vi "实验数据至图表转换.vi"() -> ()   [LabVIEW 2019]
uses:
  <vilib>/Utility/miscctls.llb/LVDateTimeRec.ctl
  <vilib>/Utility/file.llb/Read Delimited Spreadsheet (string).vi
  <vilib>/Utility/NIReport.llb/NI_report.lvclass
  <vilib>/addons/_office/NI_ReportGenerationToolkit.lvlib
  <vilib>/addons/_office/excel.llb/Excel Get Data ([str]).vi
  <vilib>/Utility/NIReport.llb/Excel/NI_Excel.lvclass
panel:
  out "时间标识":timestamp
  in  "template (empty)":path caption="模板（空）"
  out "输入+ 2":cluster{"X":dbl[], "Y":dbl[]}[](graph)
  out "电池+铜排":cluster{"X":dbl[], "Y":dbl[]}[](graph)
  in  "file path (dialog if empty)":path=path "f:/Users/black/Desktop/新建文本文档.txt"
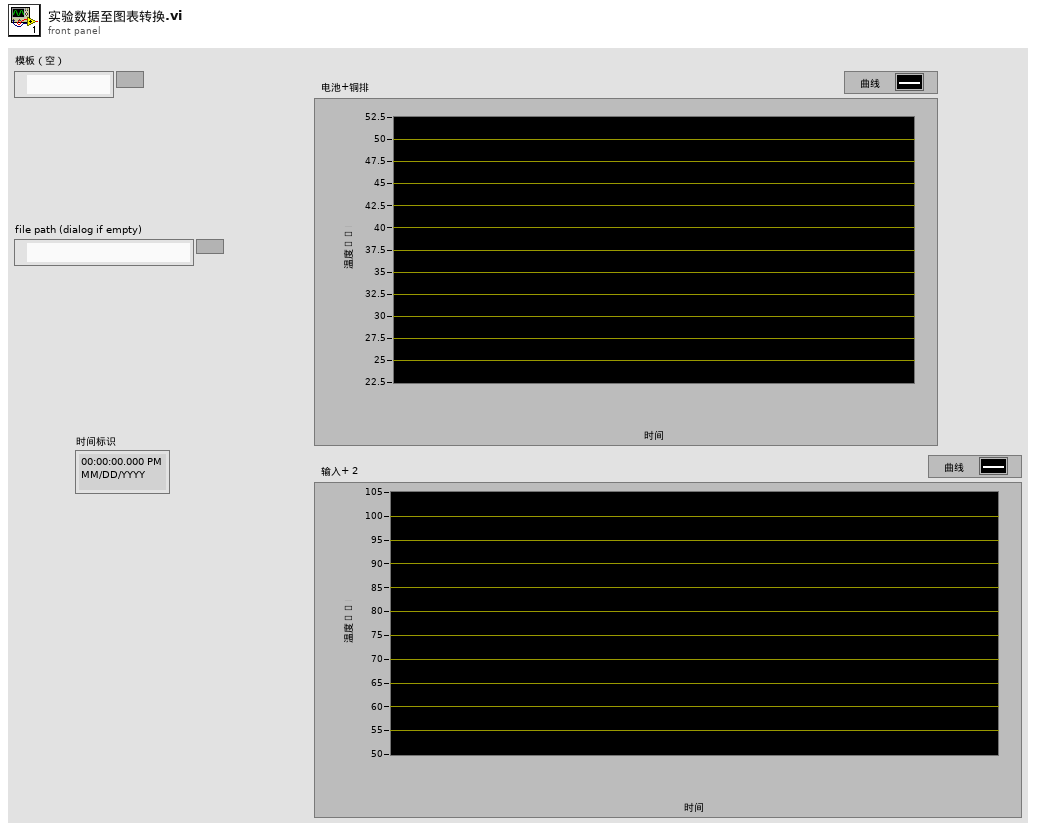
[diagram p1: front panel]
types:
  T1 = typedef "LVDateTimeRec.ctl" = cluster{"fractional second":dbl, "second":i32, "minute":i32, "hour":i32, "day of month":i32, "month":i32, "year":i32, "day of week":i32, "day of year":i32, "DST":i32}
  T2 = enum16{"Standard Report", "HTML", "Word", "Excel"}
  T3 = enum16{"maximized", "minimized", "normal", "no change"}
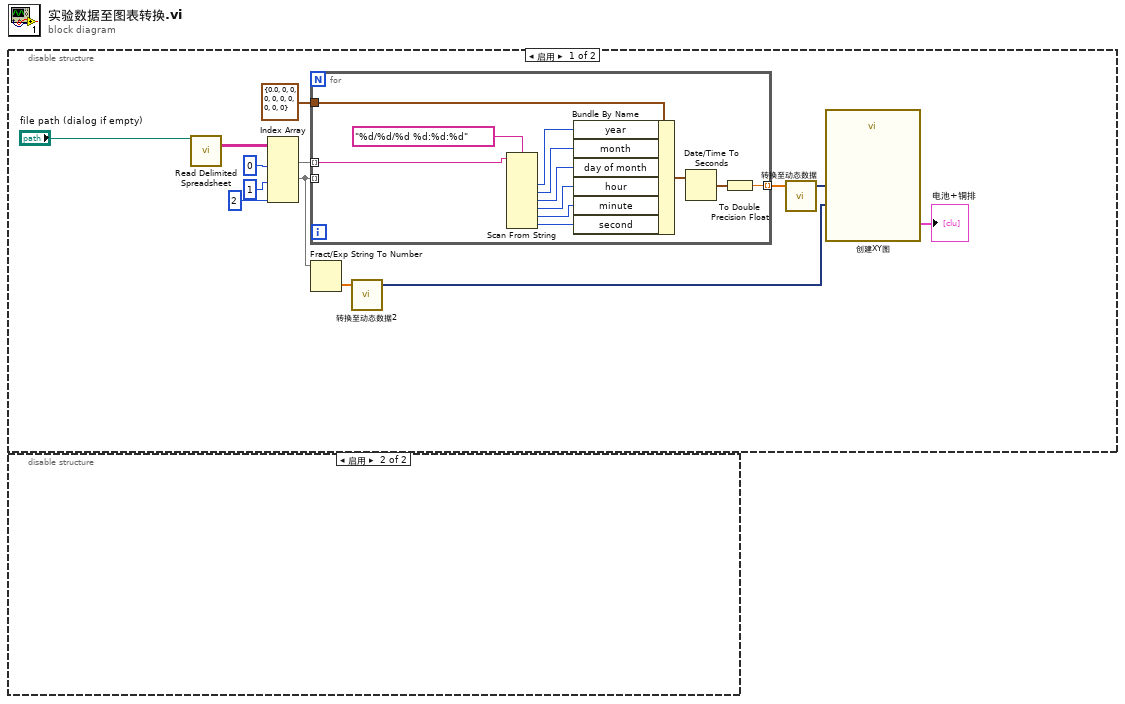
[diagram p0: block diagram]
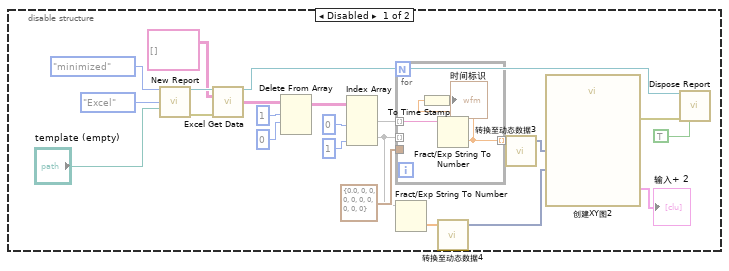
[diagram p2: hidden frame]
diagram:
  n1 = disable-structure shown="启用" {
    frame Enabled {
      n2 = call-poly <vilib>:"Read Delimited Spreadsheet.vi"("file path (dialog if empty)"="file path (dialog if empty)") -> ("all rows"=w12:string[][])  [unwired: 9 in, 5 out]
      n3 = Index Array(array=w12, index (col) #1=0 ("禁用的索引 (列)"), index (col) #2=1 ("索引 (列)"), index (col) #3=2 ("索引 (列)")) -> (element #1=w9:string[], element #2=w6:string[])  [unwired: 3 in, 1 out]
      n4 = for {
        tunnel: w9 -> [w25] mode=indexing
        tunnel: w6 -> [_] mode=indexing
        tunnel: [w15] -> w8 mode=indexing
        tunnel: T1 {"fractional second"=0.0, "second"=0, "minute"=0, "hour"=0, "day of month"=0, "month"=0, "year"=0, "day of week"=0, "day of year"=0, "DST"=0} ("输入簇") -> [w14]
        n5 = Scan From String(format string="%d/%d/%d %d:%d:%d" ("格式字符串"), input string=w25) -> (output 1=w23:i32, output 2=w22:i32, output 3=w21:i32, output 4=w20:i32, output 5=w19:i32, output 6=w18:i32)  [unwired: 8 in, 3 out]
        n6 = Bundle By Name(cluster=w14, "year"=w23, "month"=w22, "day of month"=w21, "hour"=w20, "minute"=w19, "second"=w18) -> (w17:T1)
        n7 = Date/Time To Seconds(2:w17) -> (0:w16:timestamp)  [unwired: 1 in]
        n8 = To Double Precision Float(number=w16) -> (double precision float=w15:dbl)
      }
      n9 = Fract/Exp String To Number(string=w6) -> (number=w5:dbl[])  [unwired: 3 in, 1 out]
      n10 = call "转换至动态数据2"("Array"=w5) -> ("Dynamic Data Type"=w4:dynamicdata)  [unwired: 3 in]
      n11 = call "转换至动态数据"("Array"=w8) -> ("Dynamic Data Type"=w7:dynamicdata)  [unwired: 3 in]
      n12 = call "创建XY图"("Y Input"=w4, "X Input"=w7) -> ("XY Graph"=→"电池+铜排":cluster{"X":dbl[], "Y":dbl[]}[])  [unwired: 8 in, 1 out]
    }
    frame Disabled {
    }
  }
  n13 = disable-structure shown="启用" {
    frame Disabled {
      n14 = call <vilib>:"New Report.vi"("window state (normal)"=T3."minimized", "report type"=T2."Excel", "template (empty)"="template (empty)") -> ("report out"=w46:refnum<class "NI_report.lvclass">, "error out"=w45:errorcluster)  [unwired: 11 in]
      n15 = call-poly <vilib>:"Excel Get Data.vi"("report in"=w46, "data type"=string[][] [], "error in (no error)"=w45) -> ("report out"=w33:refnum<class "NI_report.lvclass">, "data"=w29:string[][])  [unwired: 10 in, 1 out]
      n16 = Delete From Array(array=w29, length=1 ("长度"), index (row)=0 ("索引 (行)")) -> (array with subset deleted=w26:string[][])  [unwired: 1 in, 1 out]
      n17 = Index Array(array=w26, index (col) #1=0 ("禁用的索引 (列)"), index (col) #2=1 ("索引 (列)")) -> (element #1=w36:string[], element #2=w39:string[])  [unwired: 2 in]
      n18 = for {
        tunnel: w36 -> [w51] mode=indexing
        tunnel: w39 -> [_] mode=indexing
        tunnel: [w50] -> w37 mode=indexing
        tunnel: T1 {"fractional second"=0.0, "second"=0, "minute"=0, "hour"=0, "day of month"=0, "month"=0, "year"=0, "day of week"=0, "day of year"=0, "DST"=0} ("输入簇") -> [_]
        n19 = Fract/Exp String To Number(string=w51) -> (number=w50:dbl)  [unwired: 3 in, 1 out]
        n20 = To Time Stamp(1:w50) -> (0:→"时间标识":timestamp)
      }
      n21 = Fract/Exp String To Number(string=w39) -> (number=w40:dbl[])  [unwired: 3 in, 1 out]
      n22 = call "转换至动态数据4"("Array"=w40) -> ("Dynamic Data Type"=w41:dynamicdata)  [unwired: 3 in]
      n23 = call "转换至动态数据3"("Array"=w37) -> ("Dynamic Data Type"=w38:dynamicdata)  [unwired: 3 in]
      n24 = call "创建XY图2"("Y Input"=w41, "X Input"=w38) -> ("error out"=w31:errorcluster, "XY Graph"=→"输入+ 2":cluster{"X":dbl[], "Y":dbl[]}[])  [unwired: 8 in]
      n25 = call-dynamic "Dispose Report.vi"("report in"=w33, "error in (no error)"=w31, "close report? (T)"=TRUE) -> ()  [unwired: 12 in, 1 out]
    }
    frame Enabled {
    }
  }
